vi "checkout.vi"(7 "locked by?":string, 8 "error in (no error)":errorcluster) -> (0 "error out":errorcluster, 3 "GenericStimulator out":refnum<class "GenericStimulator.lvclass">)   [LabVIEW 2010, in "GenericStimulator.lvclass"]
uses:
  GenericStimulator.lvclass
  class_data.vi
  common/classes/GenericComponent/GenericComponent/GenericComponent.lvclass
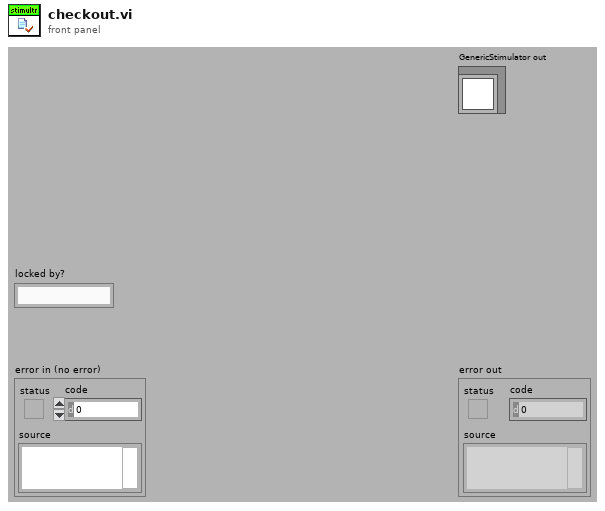
[diagram p1: front panel]
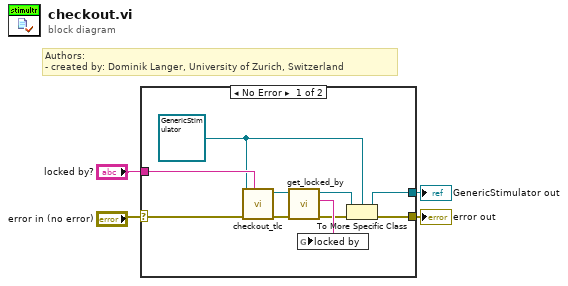
[diagram p0: block diagram]
diagram:
  # "Authors: \n- created by: Dominik Langer, University of Zurich, Switzerland"
  n1 = case shown="No Error" "error in (no error)" {
    selector: "error in (no error)" -> [w6 w15]
    tunnel: [w10 w15] -> w3
    tunnel: [w8 _] -> w2
    tunnel: "locked by?" -> [w7 _]
    frame No Error {
      w5 = refnum<class "GenericStimulator.lvclass"> refnum ("GenericStimulator.lvclass")
      n2 = call-dynamic "checkout_tlc.vi"("locked by?"=w7, "error in (no error)"=w6, "GenericToplevelComponent in"=w5) -> ("error out"=w14:errorcluster, "GenericToplevelComponent out"=w13:refnum<class "GenericToplevelComponent.lvclass">)  [unwired: 7 in]
      n3 = call "get_locked_by.vi"("error in (no error)"=w14, "GenericPlugin.lvclass in"=w13) -> ("error out"=w11:errorcluster, "locked by"=w12:string, "GenericPlugin.lvclass out"=w9:refnum<class "GenericToplevelComponent.lvclass">)  [unwired: 7 out]
      n4 = global write "class_data.vi" "locked by"(w12) -> ()
      n5 = To More Specific Class(target class=w5, reference=w9, error in=w11) -> (specific class reference=w8:refnum<class "GenericStimulator.lvclass">, error out=w10:errorcluster)
    }
    frame Error {
    }
  }
  "error out" <- w3
  "GenericStimulator out" <- w2
